vi "Pic Update Frame Image.vi"(8 "error in (no error)":errorcluster, 11 "LF2R IDE in":refnum<class "Main Panel.lvclass">) -> (0 "error out":errorcluster, 3 "LF2R IDE out":refnum<class "Main Panel.lvclass">)   [LabVIEW 2018, in "Main Panel.lvlib" / "Main Panel.lvclass"]
uses:
  Main Panel.lvclass
  Main Panel.lvclass/Main Panel.ctl
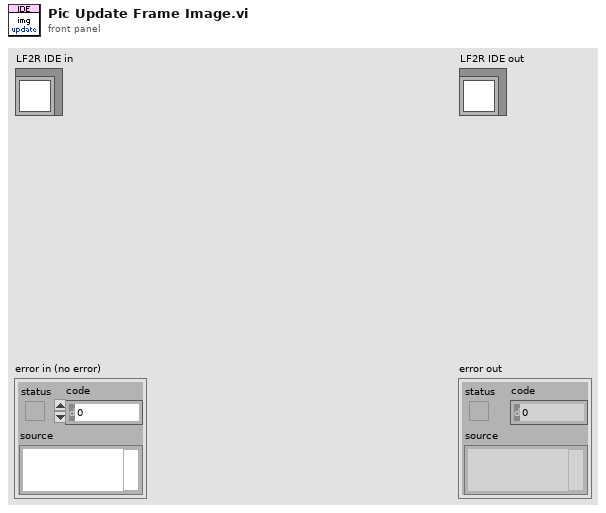
[diagram p1: front panel]
types:
  T1 = typedef "imagedata.ctl" = cluster{"image type":i32, "image depth":i32, "image":u8[], "mask":u8[], "colors":u32[], "Rectangle":cluster{"left":i16, "top":i16, "right":i16, "bottom":i16}}
  T2 = typedef "Image Json Parser.lvclass/Img Json Data.ctl" = cluster{"frames":T3[], "meta":T4}
  T3 = typedef "Image Json Parser.lvclass/Img Json Frames.ctl" = cluster{"frame":cluster{"x":i32, "y":i32, "w":i32, "h":i32}, "rotated":bool, "trimmed":bool, "spriteSourceSize":cluster{"x":i32, "y":i32, "w":i32, "h":i32}, "sourceSize":cluster{"w":i32, "h":i32}}
  T4 = typedef "Image Json Parser.lvclass/Img Json Meta.ctl" = cluster{"app":string, "version":string, "image":string, "format":string, "size":cluster{"w":i32, "h":i32}, "scale":string}
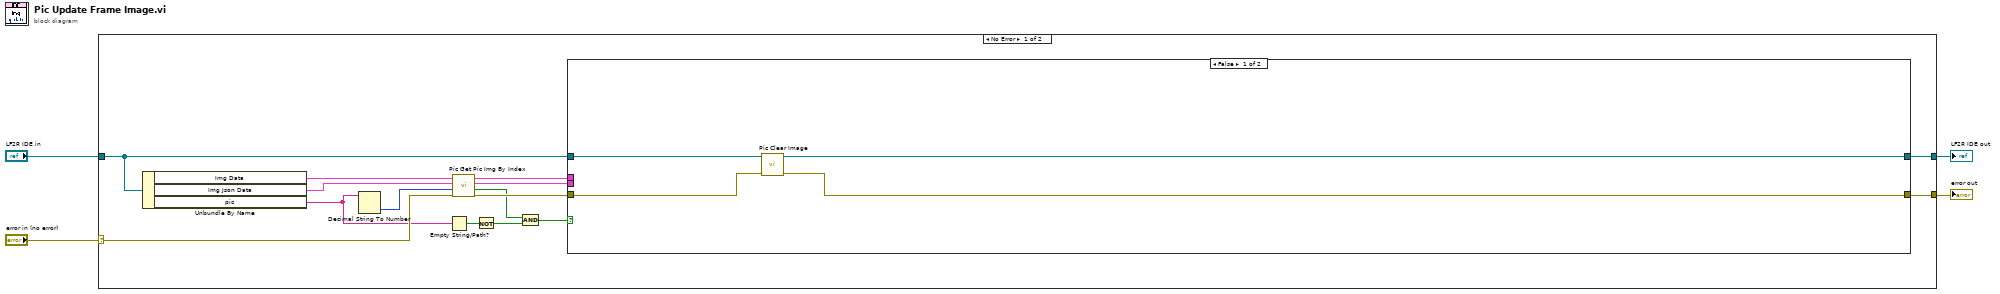
[diagram p0: block diagram]
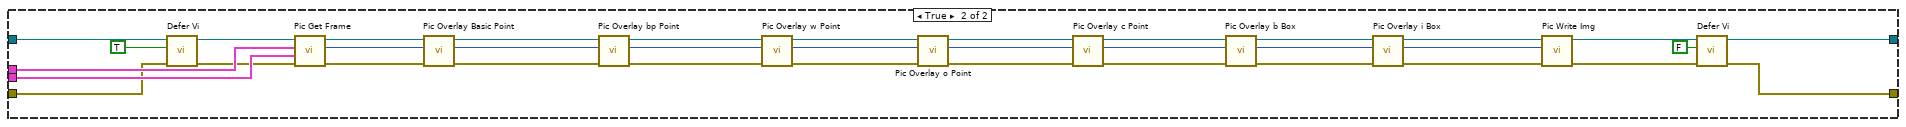
[diagram p2: hidden frame]
diagram:
  n1 = case shown="No Error" "error in (no error)" {
    selector: "error in (no error)" -> [w17 w61]
    tunnel: [w13 w61] -> w3
    tunnel: [w5 w60] -> w1
    tunnel: "LF2R IDE in" -> [w6 w60]
    frame No Error {
      n2 = Unbundle By Name(w6) -> ("Img Data"=w19:cluster{"image data":T1, "bitmap":u32[][]}[], "Img Json Data"=w18:T2[], "pic"=w11:string)
      n3 = Decimal String To Number(string=w11) -> (number=w12:i32)  [unwired: 2 in, 1 out]
      n4 = Empty String/Path?(string/path=w11) -> (empty?=w10:bool)
      n5 = call "Pic Get Pic Img By Index.vi"("error in (no error)"=w17, "Pic Num"=w12, "Img Json Data"=w18, "Img Data"=w19) -> ("error out"=w14:errorcluster, "Found?"=w8:bool, "frames"=w16:T3, "Img Data Indexed"=w15:cluster{"image data":T1, "bitmap":u32[][]})  [unwired: 4 in]
      n6 = Not(x=w10) -> (.not. x?=w9:bool)
      n7 = And(x=w8, y=w9) -> (x .and. y?=w7:bool)
      n8 = case shown="False" w7 {
        tunnel: w16 -> [_ w58]
        tunnel: w15 -> [_ w59]
        tunnel: w14 -> [w22 w28]
        tunnel: [w21 w39] -> w13
        tunnel: w6 -> [w23 w43]
        tunnel: [w20 w40] -> w5
        frame False {
          n9 = call "Pic Clear Image.vi"("error in (no error)"=w22, "LF2R IDE in"=w23) -> ("error out"=w21:errorcluster, "LF2R IDE out"=w20:refnum<class "Main Panel.lvclass">)  [unwired: 8 in]
        }
        frame True {
          n10 = call "Defer Vi.vi"("error in (no error)"=w28, "Defer Updates?"=TRUE, "Main Panel in"=w43) -> ("error out"=w25:errorcluster, "Main Panel out"=w44:refnum<class "Main Panel.lvclass">)  [unwired: 7 in]
          n11 = call "Pic Get Frame.vi"("error in (no error)"=w25, "frames"=w58, "Img Data indexed"=w59, "LF2R IDE in"=w44) -> ("error out"=w24:errorcluster, "Picture out"=w38:picture, "LF2R IDE out"=w57:refnum<class "Main Panel.lvclass">)  [unwired: 5 in]
          n12 = call "Pic Overlay Basic Point.vi"("error in (no error)"=w24, "Picture in"=w38, "LF2R IDE in"=w57) -> ("error out"=w55:errorcluster, "Picture out"=w37:picture, "LF2R IDE out"=w56:refnum<class "Main Panel.lvclass">)  [unwired: 6 in]
          n13 = call "Pic Overlay bp Point.vi"("error in (no error)"=w55, "Picture in"=w37, "LF2R IDE in"=w56) -> ("error out"=w53:errorcluster, "Picture out"=w36:picture, "LF2R IDE out"=w54:refnum<class "Main Panel.lvclass">)  [unwired: 6 in]
          n14 = call "Pic Overlay w Point.vi"("error in (no error)"=w53, "Picture in"=w36, "LF2R IDE in"=w54) -> ("error out"=w51:errorcluster, "Picture out"=w35:picture, "LF2R IDE out"=w52:refnum<class "Main Panel.lvclass">)  [unwired: 6 in]
          n15 = call "Pic Overlay o Point.vi"("error in (no error)"=w51, "Picture in"=w35, "LF2R IDE in"=w52) -> ("error out"=w49:errorcluster, "Picture out"=w34:picture, "LF2R IDE out"=w50:refnum<class "Main Panel.lvclass">)  [unwired: 6 in]
          n16 = call "Pic Overlay c Point.vi"("error in (no error)"=w49, "Picture in"=w34, "LF2R IDE in"=w50) -> ("error out"=w47:errorcluster, "Picture out"=w33:picture, "LF2R IDE out"=w48:refnum<class "Main Panel.lvclass">)  [unwired: 6 in]
          n17 = call "Pic Overlay b Box.vi"("error in (no error)"=w47, "Picture in"=w33, "LF2R IDE in"=w48) -> ("error out"=w45:errorcluster, "Picture out"=w32:picture, "LF2R IDE out"=w46:refnum<class "Main Panel.lvclass">)  [unwired: 6 in]
          n18 = call "Pic Overlay i Box.vi"("error in (no error)"=w45, "Picture in"=w32, "LF2R IDE in"=w46) -> ("error out"=w27:errorcluster, "Picture out"=w30:picture, "LF2R IDE out"=w31:refnum<class "Main Panel.lvclass">)  [unwired: 6 in]
          n19 = call "Pic Write Img.vi"("error in (no error)"=w27, "Picture"=w30, "Main Panel in"=w31) -> ("error out"=w26:errorcluster, "Main Panel out"=w29:refnum<class "Main Panel.lvclass">)  [unwired: 7 in]
          n20 = call "Defer Vi.vi"("error in (no error)"=w26, "Defer Updates?"=FALSE, "Main Panel in"=w29) -> ("error out"=w39:errorcluster, "Main Panel out"=w40:refnum<class "Main Panel.lvclass">)  [unwired: 7 in]
        }
      }
    }
    frame Error {
    }
  }
  "error out" <- w3
  "LF2R IDE out" <- w1
